vi "Construct.vi"(8 "error in (no error)":errorcluster, 11 "2D String with Headers":string[][](array[string])) -> (0 "error out":errorcluster, 3 "Table":refnum<class "SLL Table.lvclass">)   [LabVIEW 2016, in "SLL Table.lvclass"]
doc: "Constructor for the 2D Array Data"
uses:
  SLL Table.lvclass
  SLL Table.lvclass/SLL Table.ctl
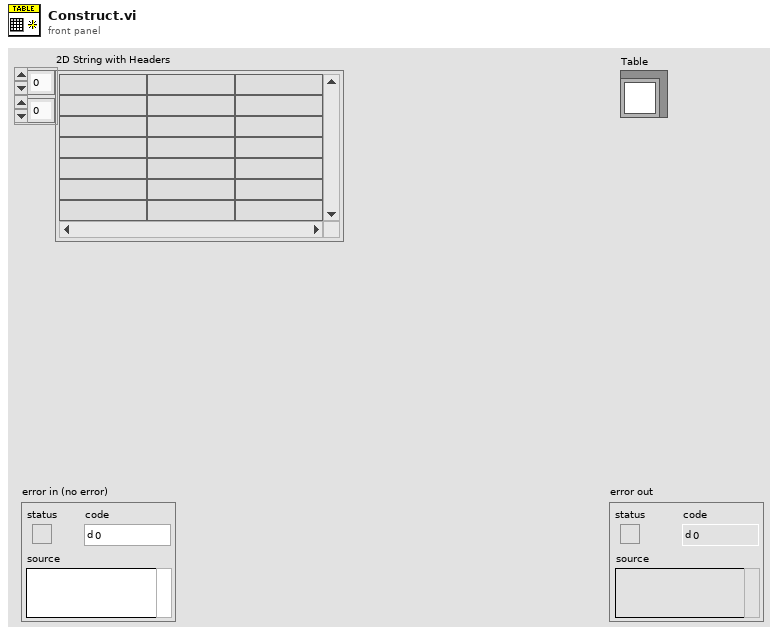
[diagram p1: front panel]
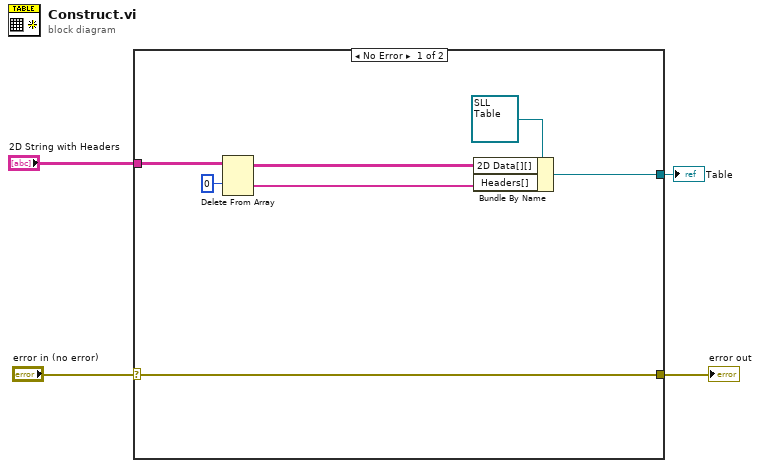
[diagram p0: block diagram]
diagram:
  n1 = case shown="No Error" "error in (no error)" {
    selector: "error in (no error)" -> [w11 w12]
    tunnel: [w11 w12] -> w4
    tunnel: "2D String with Headers" -> [w10 _]
    tunnel: [w7 _] -> w1
    frame No Error {
      n2 = Delete From Array(array=w10, index (row)=0) -> (deleted portion=w5:string[], array with subset deleted=w6:string[][])  [unwired: 2 in]
      n3 = Bundle By Name(cluster=refnum<class "SLL Table.lvclass"> refnum ("SLL Spreadsheet.lvlib:SLL Spreadsheet.lvclass"), "2D Data[][]"=w6, "Headers[]"=w5) -> (w7:refnum<class "SLL Table.lvclass">)
    }
    frame Error {
    }
  }
  "error out" <- w4
  "Table" <- w1
